vi "load_dictionary_json.vi"(7 "unit_dictionary in":variant, 8 "error in (no error)":errorcluster, 10 "symbols []":string[](array[string]), 11 "json_path":path) -> (0 "error out":errorcluster, 3 "unit_dictionary":variant)   [LabVIEW 2015, in "lv-unit-conversion.lvlib"]
doc: "load_dictionary_json can be used to load an json file into memory (it's an array of unit.ctl)."
uses:
  lv-unit-conversion.lvlib
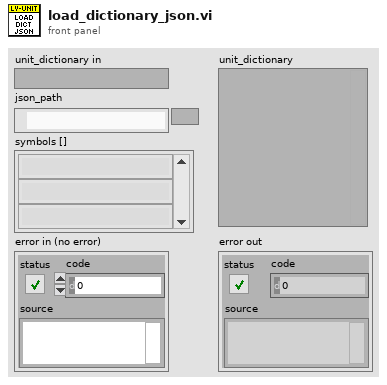
[diagram p1: front panel]
types:
  T1 = typedef "lv-unit-conversion.lvlib/unit.ctl" = cluster{"symbol":string, "name":string, "dimension":string, "is_si_unit":bool, "category":string, "base_unit":string, "conversion_reference":string, "is_exact":bool, "a":dbl, "b":dbl, "c":dbl, "d":dbl, "underlying_def":string, "description":string}
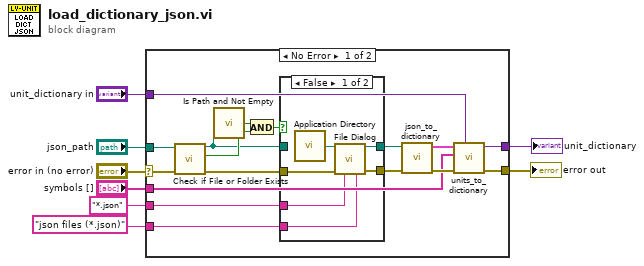
[diagram p0: block diagram]
diagram:
  n1 = case shown="No Error" "error in (no error)" {
    selector: "error in (no error)" -> [w20 w34]
    tunnel: "*.json" ("pattern (all files)") -> [w25 _]
    tunnel: "json files (*.json)" ("pattern label") -> [w24 _]
    tunnel: "json_path" -> [w21 _]
    tunnel: [w11 w34] -> w4
    tunnel: [w13 _] -> w3
    tunnel: "unit_dictionary in" -> [w10 _]
    tunnel: "symbols []" -> [w9 _]
    frame No Error {
      n2 = call <vilib>:"Check if File or Folder Exists.vi"("error in (no error)"=w20, "path"=w21) -> ("error out"=w19:errorcluster, "file or folder exists?"=w18:bool, "dup path"=w15:path)  [unwired: 7 in]
      n3 = call <vilib>:"Is Path and Not Empty.vi"("path"=w15) -> ("Is Path and Not Empty?"=w17:bool)  [unwired: 4 in]
      n4 = And(x=w17, y=w18) -> (x .and. y?=w16:bool)
      n5 = case shown="False" w16 {
        tunnel: w25 -> [w31 _]
        tunnel: w24 -> [w30 _]
        tunnel: [w29 w33] -> w23
        tunnel: [w28 w32] -> w22
        tunnel: w19 -> [w27 w32]
        tunnel: w15 -> [_ w33]
        frame False {
          n6 = call <vilib>:"Application Directory.vi"() -> ("Application Directory"=w26:path)
          n7 = call "File Dialog"("start path"=w26, "error in"=w27, "pattern (all files)"=w31, "pattern label"=w30) -> ("selected path"=w29:path, "error out"=w28:errorcluster)  [unwired: 8 in, 2 out]
        }
        frame True {
        }
      }
      n8 = call "json_to_dictionary.vi"("error in (no error)"=w22, "json_path"=w23) -> ("error out"=w12:errorcluster, "units []"=w14:T1[])  [unwired: 8 in]
      n9 = call "units_to_dictionary.vi"("unit_dictionary in"=w10, "error in (no error)"=w12, "symbols []"=w9, "units []"=w14) -> ("error out"=w11:errorcluster, "unit_dictionary out"=w13:variant)  [unwired: 6 in]
    }
    frame Error {
    }
  }
  "error out" <- w4
  "unit_dictionary" <- w3
